vi "FileUtil_DefaultDir.vi"(11 "Path in":path) -> (3 "Path Out":path)   [LabVIEW 2019, in "Trajectory_Library.lvlib"]
doc: "If given path is relative insert the default data directory. If given path is absolute, pass it through unchanged. The resulting path is always absolute."
uses:
  Trajectory_Library.lvlib
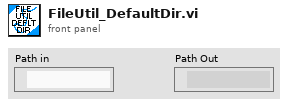
[diagram p1: front panel]
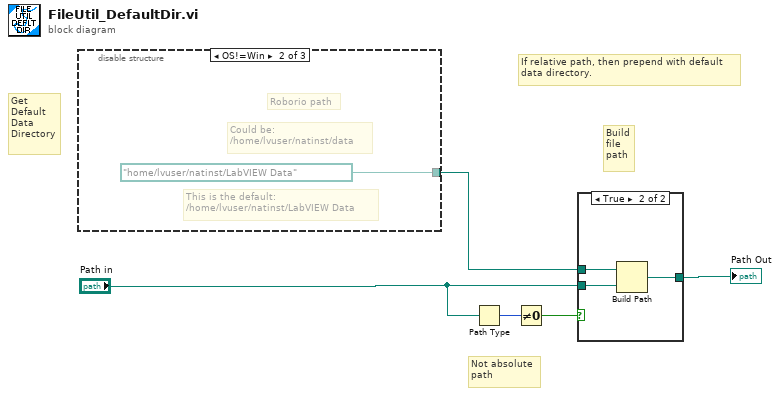
[diagram p0: block diagram]
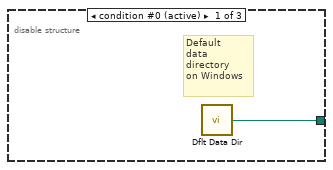
[diagram p3: hidden frame]
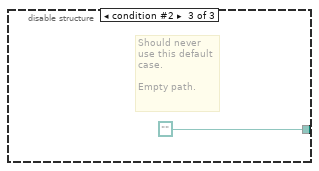
[diagram p4: hidden frame]
diagram:
  # "If relative path, then prepend with default\ndata directory."
  # "Not absolute\npath"
  # "Get\nDefault\nData\nDirectory"
  # "Build\nfile\npath"
  n1 = disable-structure shown="OS!=Win" {
    disable-tunnel: [w6 path "/home/lvuser/natinst/LabVIEW Data" path ""] -> w1
    frame condition #0 (active) {
      # "Default\ndata\ndirectory\non Windows"
      n2 = call <vilib>:"Dflt Data Dir.vi"() -> ("App:Default Data Directory"=w6:path)
    }
    frame condition #1 {
      # "This is the default:\n/home/lvuser/natinst/LabVIEW Data"
      # "Could be:\n/home/lvuser/natinst/data"
      # "Roborio path"
    }
    frame condition #2 {
      # "Should never\nuse this default\ncase.\n\nEmpty path."
    }
  }
  n3 = Path Type(1:"Path in") -> (0:w2:i16)
  n4 = Not Equal To 0?(x=w2) -> (x != 0?=w3:bool)
  n5 = case shown="True" w3 {
    tunnel: [w9 w12] -> w4
    tunnel: w1 -> [_ w11]
    tunnel: "Path in" -> [w9 w10]
    frame False {
    }
    frame True {
      n6 = Build Path(base path=w11, name or relative path=w10) -> (appended path=w12:path)
    }
  }
  "Path Out" <- w4
